vi "CALC AUTO DRIVE TIMES.vi"(8 "error in (no error)":errorcluster, 10 "throttle VBus":dbl=0.65, 11 "desired distance (ft)":dbl) -> (0 "error out":errorcluster, 1 "velocity\n(ft/s)":dbl, 2 "throttle out":dbl=0.65, 3 "Milliseconds":u16)   [LabVIEW 2023]
uses:
  ctrl defs/ctrl MOTOR SELECT.ctl
  Global odometry.vi
  Global INIT.vi
  <vilib>/Rock Robotics/WPI/ThirdParty/JAS_Junk/TrajLib/Trajectory_Library.lvlib
panel:
  out "NORMAL.DRIVE":dbl
  out "velocity\n(in/s)":dbl
  out "max velocity\n(in/s)":dbl
  out "max speed\n(rpm)":dbl
  out "theoretical\nfree speed (rpm)":dbl
  out "gear ratio":dbl
  out "MOTOR SELECT":T1 items=["REV NEO"=5676, "REV NEO 550"=11000, "VEX Falcon"=6380, "WC Kraken"=6000]
  out "wheel\ncircumference (in)":dbl
  out "efficiency":dbl=0.5942
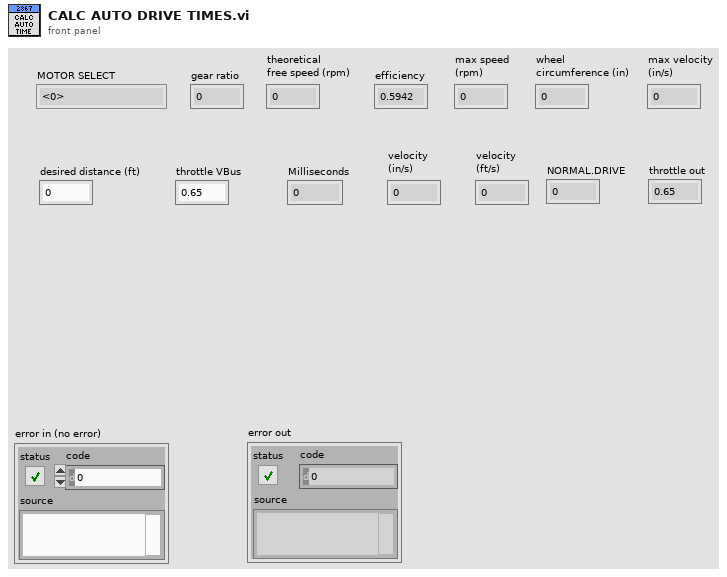
[diagram p1: front panel]
types:
  T1 = typedef "ctrl MOTOR SELECT.ctl" = i16
  T2 = typedef "ctrl swerve motor.ctl" = cluster{"description":string, "MOTOR SELECT":T1, "Installed?":bool, "CAN ID":u8, "refnum name":string, "Invert":bool, "Idle Mode":T3, "Current limiting":T4, "MOTOR PIDF coefficients":T5, "gear ratio":dbl}
  T3 = typedef "Spark MAX Idle Mode.ctl" = enum16{"Coast", "Brake"}
  T4 = typedef "ctrl Spark MAX current limiting.ctl" = cluster{"Linearized":bool, "Free Speed (A)":dbl, "Primay (A)":dbl, "Limit RPM (0)":u32}
  T5 = typedef "ctrl motor PIDF coefficients.ctl" = cluster{"PIDF":cluster{"P Gain":dbl, "I Gain":dbl, "D Gain":dbl, "F Gain":dbl, "I Zone":dbl, "Min Output":dbl, "Max Output":dbl}, "Smart Motion":T6}
  T6 = typedef "Spark MAX Smart Motion Parameters.ctl" = cluster{"Max Velocity":dbl, "Max Acceleration":dbl, "Minimum Velocity Output":dbl, "Allowed Closed Loop Error":dbl}
  T7 = typedef "ctrl swerve speeds.ctl" = cluster{"NORMAL":cluster{"DRIVE":dbl, "STEER":dbl}, "TURTLE":cluster{"DRIVE":dbl, "STEER":dbl}, "TURBO":cluster{"DRIVE":dbl, "STEER":dbl}}
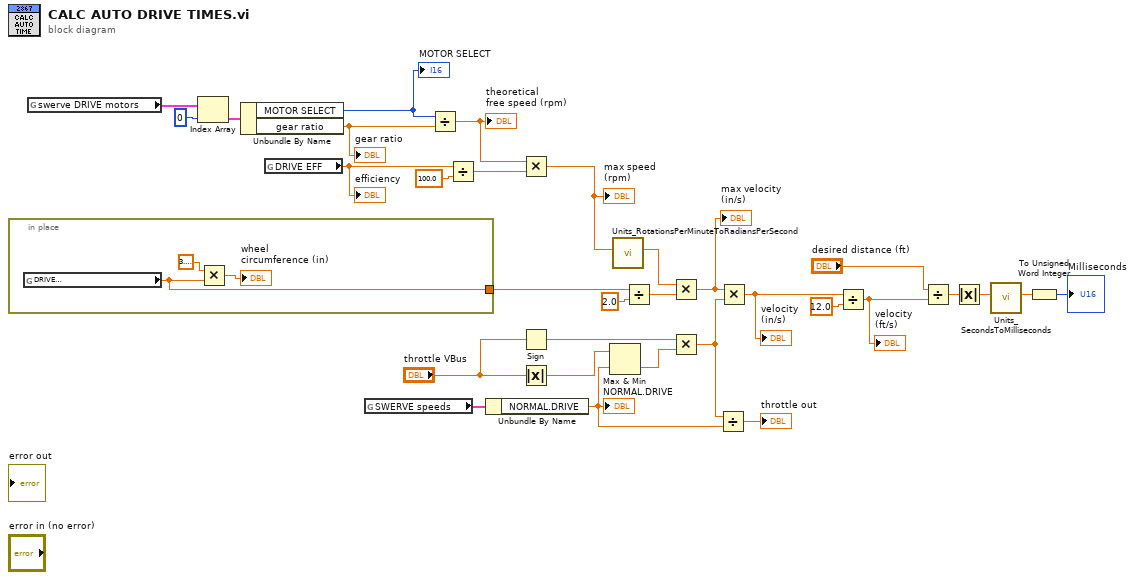
[diagram p0: block diagram]
diagram:
  n1 = in-place {
    in-place-border: [w32] -> w23
    n2 = global read "Global INIT.vi" "DRIVE\nwheel diam (in)"() -> (w32:dbl)
    n3 = Multiply(x=3.141592653589793, y=w32) -> (x*y=→"wheel\ncircumference (in)":dbl)
  }
  n4 = global read "Global INIT.vi" "swerve DRIVE motors"() -> (w31:T2[])
  n5 = Index Array(array=w31, index=0) -> (element=w29:T2)
  n6 = Unbundle By Name(w29) -> ("MOTOR SELECT"=w28:T1, "gear ratio"=w27:dbl)
  "MOTOR SELECT" <- w28
  "gear ratio" <- w27
  n7 = global read "Global odometry.vi" "DRIVE EFF"() -> (w12:dbl)
  "efficiency" <- w12
  n8 = global read "Global odometry.vi" "SWERVE speeds"() -> (w9:T7)
  n9 = Divide(x=w28, y=w27) -> (x/y=w26:dbl)
  "theoretical\nfree speed (rpm)" <- w26
  n10 = Divide(x=w12, y=100.0) -> (x/y=w13:dbl)
  n11 = Unbundle By Name(w9) -> ("NORMAL.DRIVE"=w7:dbl)
  "NORMAL.DRIVE" <- w7
  n12 = Multiply(x=w26, y=w13) -> (x*y=w25:dbl)
  "max speed\n(rpm)" <- w25
  n13 = Sign(1:"throttle VBus") -> (0:w4:dbl)
  n14 = Absolute Value(x="throttle VBus") -> (abs(x)=w6:dbl)
  n15 = Max & Min(x=w6, y=w7) -> (min(x,y)=w3:dbl)  [unwired: 1 out]
  n16 = call <vilib>:"Units_RotationsPerMinuteToRadiansPerSecond.vi"("RotationsPerMinute"=w25) -> ("RadiansPerSecond"=w24:dbl)  [unwired: 10 in]
  n17 = Divide(x=w23, y=2.0) -> (x/y=w22:dbl)
  n18 = Multiply(x=w24, y=w22) -> (x*y=w20:dbl)
  "max velocity\n(in/s)" <- w20
  n19 = Multiply(x=w4, y=w3) -> (x*y=w2:dbl)
  n20 = Divide(x=w2, y=w7) -> (x/y=→"throttle out":dbl)
  n21 = Multiply(x=w20, y=w2) -> (x*y=w19:dbl)
  "velocity\n(in/s)" <- w19
  n22 = Divide(x=w19, y=12.0) -> (x/y=w16:dbl)
  "velocity\n(ft/s)" <- w16
  n23 = Divide(x="desired distance (ft)", y=w16) -> (x/y=w15:dbl)
  n24 = Absolute Value(x=w15) -> (abs(x)=w1:dbl)
  n25 = call <vilib>:"Units_SecondsToMilliseconds.vi"("Seconds"=w1) -> ("Milliseconds"=w14:dbl)  [unwired: 10 in]
  n26 = To Unsigned Word Integer(number=w14) -> (unsigned 16bit integer=→"Milliseconds":u16)
